vi "Create Virtual Axis (by Ratio).vi"(6 "Axis Numbers (1,2)":u8[](array[numeric])=[1, 2], 7 "Ratio":i32[](array[numeric]), 8 "error in (no error)":errorcluster, 9 "Device Number":string, 10 "Virtual Axis Number (1)":u8=1, 11 "VISA resource name":refnum<visa-resource-name>) -> (0 "error out":errorcluster, 3 "VISA resource name out":refnum<visa-resource-name>)   [LabVIEW 2013, in "Zaber A Series.lvlib"]
doc: "Configured a virtual axis on a device that supports it. A virtual axis defines an angular relationship between two axes such that when the virtual axis is moved, both axes move in proportion to the angle. Normal single-axis move commands can still be used while a virtual axis is configured, but will only move one axis at a time.\n\nTo configure a virtual axis you must specify an identifying number for it, between 1 and the value of the \"virtual.numvirtual\" device setting. You must also specify two axis numbers to be members of the group, and the relative movement ratios of the axes. The ratio numbers are signed integers that can each be between -2147483648 and 2147483648. Their proportion controls the relative movement speeds of the physical axes and their sign controls the directions. There must be one ratio entry for each physical axis comprising the virtual axis.\n\nTo use the features of a virtual axis you must use the virtual axis specific VIs provided.\n\nThis VI does not check in advance for error conditions such as lockstep not being supported on the device or no virtual axis numbers being available.\n\nThis VI requires that the Initialize VI has been called with the same serial port."
uses:
  Zaber A Series.lvlib
  Private/All Commands.ctl
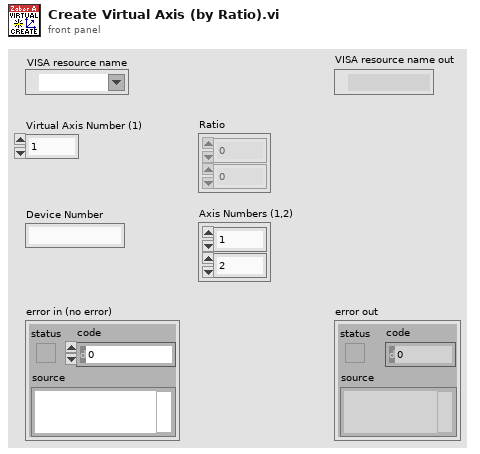
[diagram p1: front panel]
types:
  T1 = typedef "Zaber A Series.lvlib/All Commands.ctl" = string
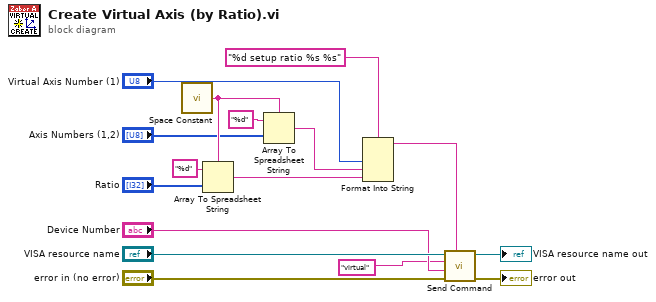
[diagram p0: block diagram]
diagram:
  n1 = call <vilib>:"Space Constant.vi"() -> ("String"=w11:string)
  n2 = Array To Spreadsheet String(delimiter (Tab)=w11, array="Ratio", 3:"%d" ("format string")) -> (spreadsheet string=w4:string)
  n3 = Array To Spreadsheet String(delimiter (Tab)=w11, array="Axis Numbers (1,2)", 3:"%d" ("format string")) -> (spreadsheet string=w5:string)
  n4 = Format Into String(format string="%d setup ratio %s %s", "Virtual Axis Number (1)", w5, w4) -> (resulting string=w3:string)  [unwired: 2 in, 1 out]
  n5 = call "Send Command.vi"("Data"=w3, "error in (no error)"="error in (no error)", "Device and Axis"="Device Number", "Command"=T1 "virtual" ("Complete Command List"), "VISA resource name"="VISA resource name") -> ("error out"=→"error out":errorcluster, "VISA resource name out"=→"VISA resource name out":refnum<visa-resource-name>)  [unwired: 1 in, 4 out]
